vi "readInTimeLabel.vi"(8 "error in (no error)":errorcluster, 10 "eventXML":refnum<k20>, 11 "Delay in":refnum<class "Delay.lvclass">) -> (0 "error out":errorcluster, 2 "eventXML out":refnum<k20>, 3 "Delay out":refnum<class "Delay.lvclass">)   [LabVIEW 2009, in "Tools.lvlib" / "Scripting.lvlib" / "Delay.lvclass"]
uses:
  Delay.lvclass
  <vilib>/xml/Close Reference(NNMap).vi
  <vilib>/xml/Close Reference(Node).vi
  Delay.lvclass/Delay.ctl
  Program Files/National Instruments/LabVIEW 2009/resource/objmgr/DOMUserDefRef.rc
  <vilib>/xml/NI_XML.lvlib
  ScriptEvent.lvclass
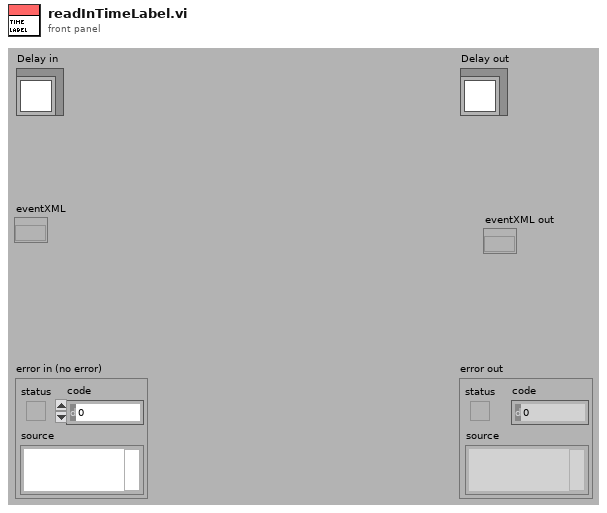
[diagram p1: front panel]
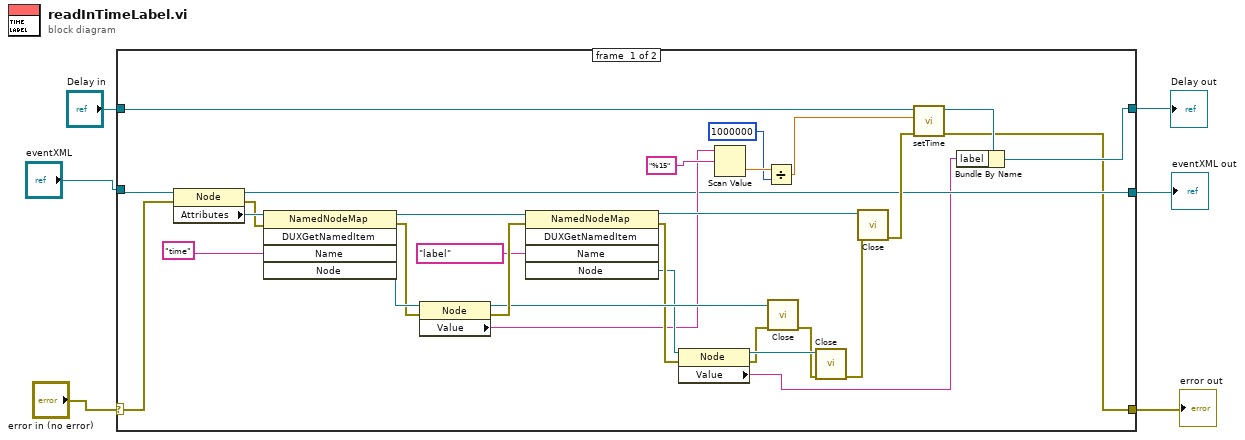
[diagram p0: block diagram]
diagram:
  n1 = case shown="No Error" "error in (no error)" {
    selector: "error in (no error)" -> [w14 w38]
    tunnel: [w8 w38] -> w1
    tunnel: [w9 w37] -> w6
    tunnel: "Delay in" -> [w15 w37]
    tunnel: "eventXML" -> [w36 _]
    tunnel: [w11 _] -> w2
    frame #0 {
      n2 = property class="Node"(reference=w36, error in=w14) -> (reference out=w11:refnum<k20>, error out=w32:errorcluster, "Attributes"=w33:refnum<k20>)
      n3 = invoke class="NamedNodeMap" method="DUXGetNamedItem"(reference=w33, error in=w32, "Name"="time") -> (reference out=w31:refnum<k20>, error out=w34:errorcluster, "Node"=w35:refnum<k20>)  [unwired: 2 in, 2 out]
      n4 = property class="Node"(reference=w35, error in=w34) -> (reference out=w29:refnum<k20>, error out=w30:errorcluster, "Value"=w18:string)
      n5 = invoke class="NamedNodeMap" method="DUXGetNamedItem"(reference=w31, error in=w30, "Name"="label") -> (reference out=w24:refnum<k20>, error out=w23:errorcluster, "Node"=w22:refnum<k20>)  [unwired: 2 in, 2 out]
      n6 = property class="Node"(reference=w22, error in=w23) -> (reference out=w28:refnum<k20>, error out=w27:errorcluster, "Value"=w7:string)
      n7 = Scan Value(string=w18, format string="%15") -> (value=w17:dbl)  [unwired: 1 in, 1 out]
      n8 = Divide(x=w17, y=1000000) -> (x/y=w13:dbl)
      n9 = call-poly <vilib>:"Close.vi"("error in (no error)"=w27, "node"=w29) -> ("error out"=w26:errorcluster)  [unwired: 7 in]
      n10 = call-poly <vilib>:"Close.vi"("error in (no error)"=w26, "node"=w28) -> ("error out"=w25:errorcluster)  [unwired: 7 in]
      n11 = call-poly <vilib>:"Close.vi"("error in (no error)"=w25, "named node map"=w24) -> ("error out"=w12:errorcluster)  [unwired: 7 in]
      n12 = call "setTime.vi"("error in (no error)"=w12, "time"=w13, "ScriptEvent.lvclass in"=w15) -> ("error out"=w8:errorcluster, "ScriptEvent.lvclass out"=w10:refnum<class "Delay.lvclass">)  [unwired: 7 in]
      n13 = Bundle By Name(cluster=w10, "label"=w7) -> (w9:refnum<class "Delay.lvclass">)
    }
    frame #1 {
    }
  }
  "error out" <- w1
  "Delay out" <- w6
  "eventXML out" <- w2
